vi "userinterfaceassignment1.vi"() -> ()   [LabVIEW 2019]
uses:
  <vilib>/Utility/file.llb/Read Delimited Spreadsheet (string).vi
panel:
  out "?":bool
  out "max value":i16
  out "x .and. y?":i16[][](array[numeric])
  out "numerical array2":i16[][](array[numeric])
  out "numerical array 1":i16[][](array[numeric])
  out "PW":bool[][](array[boolean])
  in  "password":string
  out "UN":bool[][](array[boolean])
  in  "UserName":string
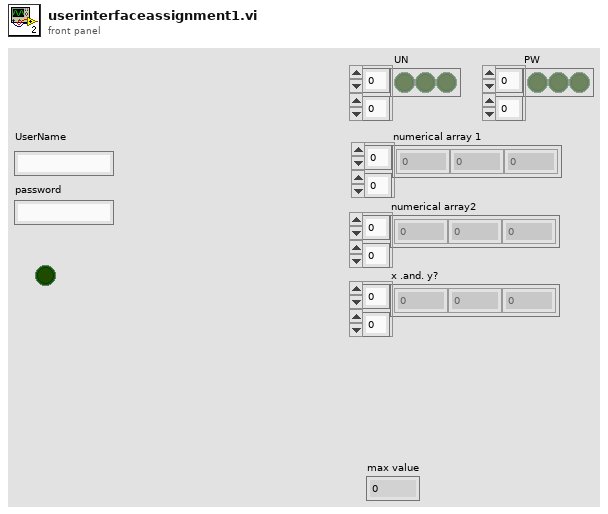
[diagram p1: front panel]
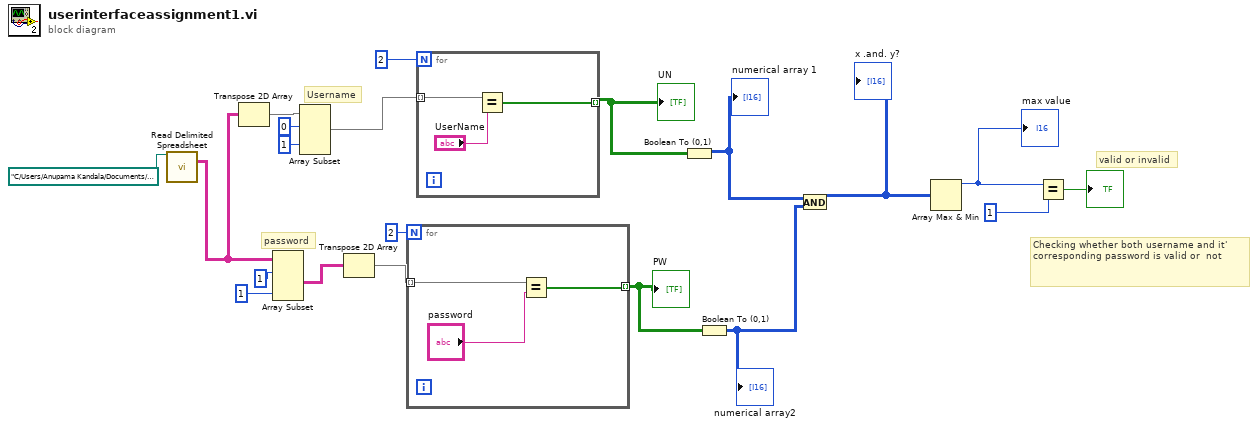
[diagram p0: block diagram]
diagram:
  # "Checking whether both username and it'\ncorresponding password is valid or  not"
  # "valid or invalid"
  # "password"
  # "Username"
  n1 = call-poly <vilib>:"Read Delimited Spreadsheet.vi"("file path (dialog if empty)"=path "C:/Users/Anupama Kandala/Documents/LabVIEW folders/database.xls") -> ("all rows"=w17:string[][])  [unwired: 9 in, 5 out]
  n2 = Transpose 2D Array(2D array=w17) -> (transposed array=w16:string[][])
  n3 = Array Subset(array=w17, index (row)=1 ("index"), index (col)=1 ("index")) -> (w10:string[][])  [unwired: 2 in]
  n4 = Array Subset(array=w16, index (row)=0 ("index"), index (col)=1 ("index")) -> (w13:string[][])  [unwired: 2 in]
  n5 = Transpose 2D Array(2D array=w10) -> (transposed array=w9:string[][])
  n6 = for {
    N: 2 -> [_]
    tunnel: w9 -> [w23] mode=indexing
    tunnel: [w21] -> w7 mode=indexing
    n7 = Equal?(x=w23, y="password") -> (x = y?=w21:bool[])
  }
  "PW" <- w7
  n8 = for {
    N: 2 -> [_]
    tunnel: w13 -> [w25] mode=indexing
    tunnel: [w24] -> w8 mode=indexing
    n9 = Equal?(x=w25, y="UserName") -> (x = y?=w24:bool[])
  }
  "UN" <- w8
  n10 = Boolean To (0,1)(Boolean=w8) -> (0, 1=w6:i16[][])
  "numerical array 1" <- w6
  n11 = Boolean To (0,1)(Boolean=w7) -> (0, 1=w5:i16[][])
  "numerical array2" <- w5
  n12 = And(x=w6, y=w5) -> (x .and. y?=w4:i16[][])
  "x .and. y?" <- w4
  n13 = Array Max & Min(array=w4) -> (max value=w3:i16)  [unwired: 3 out]
  "max value" <- w3
  n14 = Equal?(x=w3, y=1) -> (x = y?=→"?":bool)
